vi "Read TypeMap.vi"(8 "error in (no error)":errorcluster, 11 "object in":refnum<class>) -> (0 "error out":errorcluster, 1 "found/replaced?":bool, 2 "TypeMap in":refnum<class "TypeMap.lvclass">, 3 "object out":refnum<class>)   [LabVIEW 2020, in "ORM.lvlib" / "TypeMap.lvclass"]
uses:
  TypeMap.lvclass
  TypeMap.lvclass/TypeMap.ctl
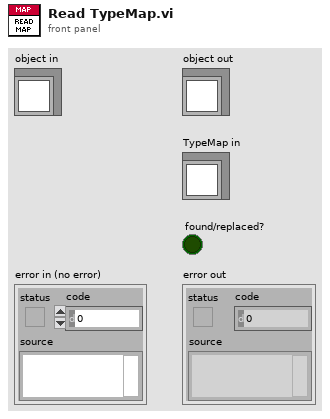
[diagram p1: front panel]
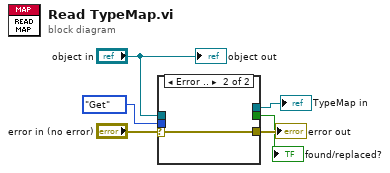
[diagram p0: block diagram]
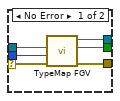
[diagram p2: hidden frame]
diagram:
  n1 = case shown="Error .." "error in (no error)" {
    selector: "error in (no error)" -> [w10 w13]
    tunnel: "object in" -> [w12 _]
    tunnel: enum16{"Get", "Set"}."Get" ("Action") -> [w11 _]
    tunnel: [w9 w13] -> w3
    tunnel: [w8 _] -> w2
    tunnel: [w7 _] -> w1
    frame No Error {
      n2 = call "TypeMap FGV.vi"("error in (no error)"=w10, "Action"=w11, "object"=w12) -> ("error out"=w9:errorcluster, "found/replaced?"=w7:bool, "TypeMap out"=w8:refnum<class "TypeMap.lvclass">)  [unwired: 6 in]
    }
    frame Error {
    }
  }
  "error out" <- w3
  "TypeMap in" <- w2
  "found/replaced?" <- w1
  "object out" <- "object in"
